vi "Decrypt.vi"(8 "error in (no error)":errorcluster, 10 "Message":string, 11 "FFT in":refnum<class "FFT.lvclass">) -> (0 "error out":errorcluster, 2 "Decrypted Message":string, 3 "FFT out":refnum<class "FFT.lvclass">)   [LabVIEW 2019, in "TSC Event Logger.lvlib" / "FFT.lvclass"]
doc: "The decrypt method will taken an encrypted message in and return a decrypted string output.\n\n<b>Code Developed By:</b>\nTechnology Service Corporation\nBloomington, IN 47403\nwww.tsc.com/atcs\n\nDeveloper:\nDaniel Coons"
uses:
  FFT.lvclass
  C:/Development/Open Source/tsc-event-logger/Encryption/Encryption.lvclass
  Encryption.lvclass/Encryption.ctl
  <vilib>/Analysis/2dsp.llb/Inverse Real FFT.vi
  Read SALT.vi
  Read Multiplier.vi
  <vilib>/regexp/Match Regular Expression.xnode
  <vilib>/Analysis/NI_AALPro.lvlib
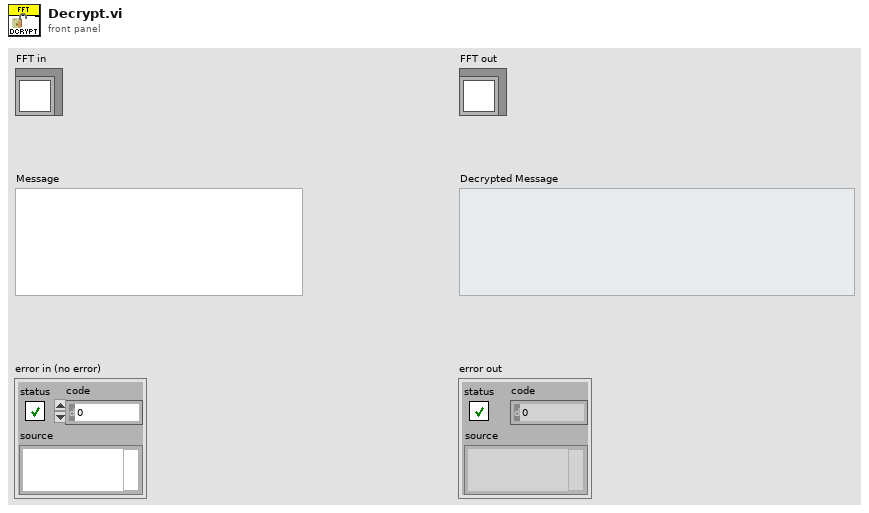
[diagram p1: front panel]
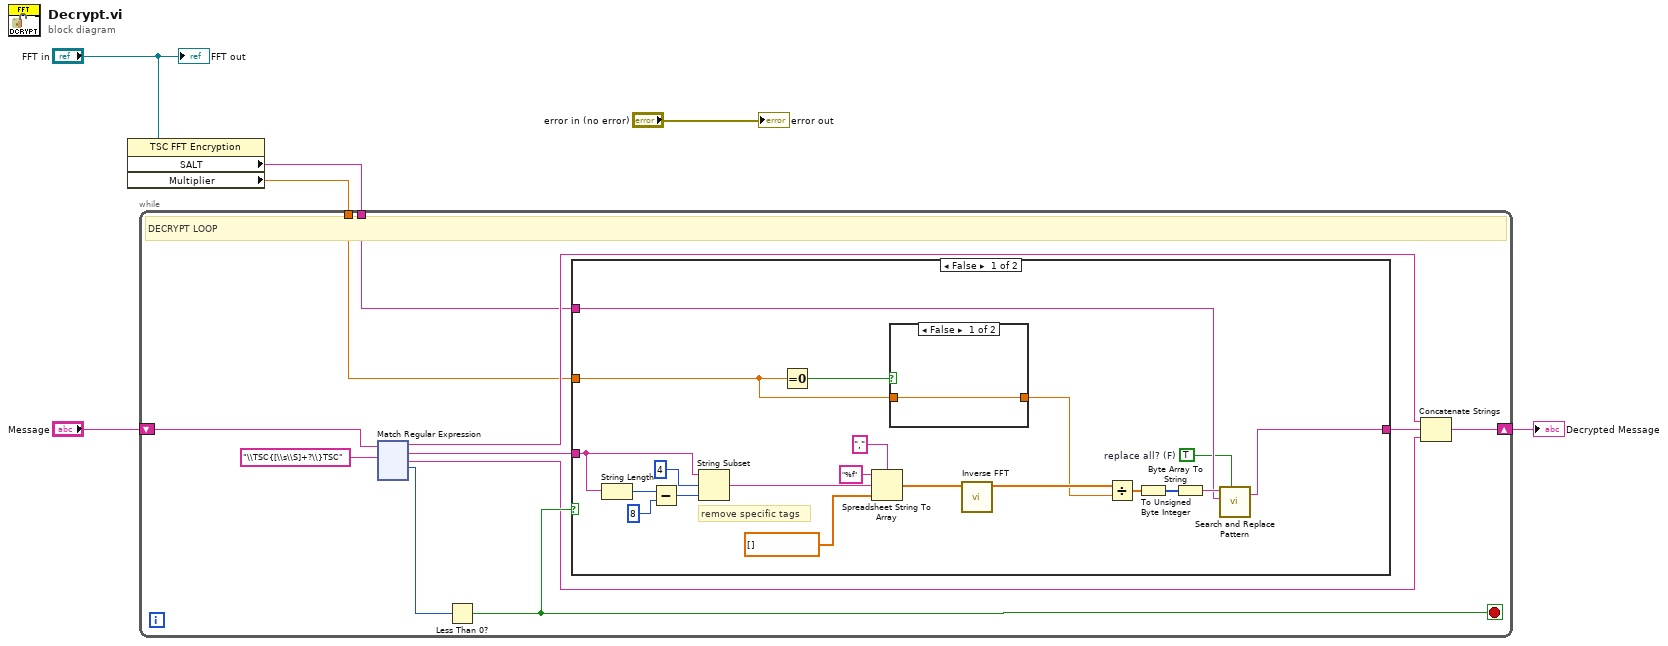
[diagram p0: block diagram]
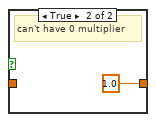
[diagram p2: hidden frame]
diagram:
  n1 = property class="TSC FFT Encryption"(reference="FFT in") -> ("SALT"=w1:string, "Multiplier"=w2:dbl)  [unwired: 1 in, 2 out]
  n2 = while {
    shift-right: [w11] -> w4
    shift-left: "Message" -> [w16]
    tunnel: w2 -> [w8]
    tunnel: w1 -> [w7]
    stop <- w14 stop-if-true
    # "DECRYPT LOOP"
    n3 = xnode "Match Regular Expression"("input string"=w16, "regular expression"="\\TSC{[\\s\\S]+?\\}TSC") -> ("before match"=w10:string, "whole match"=w13:string, "after match"=w9:string, "offset past match"=w15:i32)  [unwired: 4 in, 1 out]
    n4 = Less Than 0?(x=w15) -> (x < 0?=w14:bool)
    n5 = case shown="False" w14 {
      tunnel: w13 -> [w36 _]
      tunnel: [w18 _] -> w12
      tunnel: w8 -> [w26 _]
      tunnel: w7 -> [w20 _]
      frame False {
        w19 = TRUE  # replace all? (F)
        # "remove specific tags"
        n6 = String Length(string=w36) -> (length=w35:i32)
        n7 = Subtract(x=w35, y=8 ("x")) -> (x-y=w34:i32)
        n8 = String Subset(string=w36, offset (0)=4, length (rest)=w34) -> (substring=w32:string)
        n9 = Equal To 0?(x=w26) -> (x = 0?=w27:bool)
        n10 = Spreadsheet String To Array(delimiter (Tab)=",", format string="%f", spreadsheet string=w32, array type (2D Dbl)=cdb[] []) -> (array=w28:cdb[])
        n11 = case shown="False" w27 {
          tunnel: w26 -> [w38 _]
          tunnel: [w38 1.0 ("Multiplier")] -> w24
          frame False {
          }
          frame True {
            # "can't have 0 multiplier"
          }
        }
        n12 = call-poly <vilib>:"Inverse FFT.vi"("FFT {X}"=w28) -> ("X"=w25:dbl[])  [unwired: 9 in, 1 out]
        n13 = Divide(x=w25, y=w24) -> (x/y=w22:dbl[])
        n14 = To Unsigned Byte Integer(number=w22) -> (unsigned 8bit integer=w23:u8[])
        n15 = Byte Array To String(unsigned byte array=w23) -> (string=w21:string)
        n16 = call <vilib>:"Search and Replace Pattern.vi"("string"=w21, "regular expression (\"\")"=w20, "replace all? (F)"=w19) -> ("result string"=w18:string)  [unwired: 2 in, 1 out]
      }
      frame True {
      }
    }
    n17 = Concatenate Strings(w10, w12, w9) -> (w11:string)
  }
  "Decrypted Message" <- w4
  "error out" <- "error in (no error)"
  "FFT out" <- "FFT in"
